vi "通知路由使用时间结束.vi"(7 "ACOM":string="A%d:COM%d", 11 "RF_Now":T1) -> ()   [LabVIEW 2011]
uses:
  Global/SeverGlobal.vi
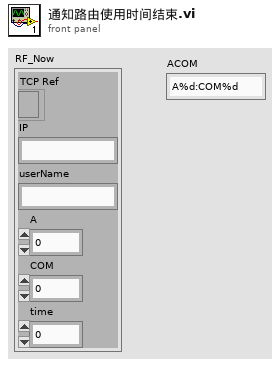
[diagram p1: front panel]
types:
  T1 = cluster{"TCP Ref":refnum<k5>, "IP":string, "userName":string, "A":u16, "COM":u16, "time":u32}
  T2 = cluster{"TCP Ref":refnum<k5>, "Broadcast":refnum<k5>, "IP":string, "port":u16, "userName":string, "passWord":string, "authority":string}[]
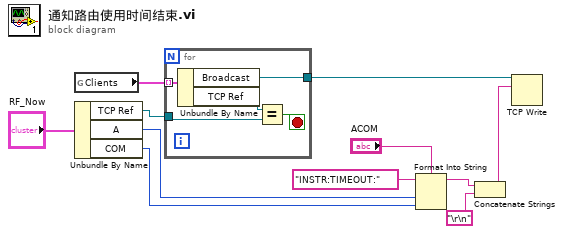
[diagram p0: block diagram]
diagram:
  n1 = global read "SeverGlobal.vi" "Clients"() -> (w9:T2)
  n2 = Unbundle By Name("RF_Now") -> ("TCP Ref"=w10:refnum<k5>, "A"=w2:u16, "COM"=w1:u16)
  n3 = for {
    tunnel: w9 -> [w16] mode=indexing
    tunnel: w10 -> [w14]
    tunnel: [w12] -> w11
    stop <- w13 stop-if-true
    n4 = Unbundle By Name(w16) -> ("Broadcast"=w12:refnum<k5>, "TCP Ref"=w15:refnum<k5>)
    n5 = Equal?(x=w15, y=w14) -> (x = y?=w13:bool)
  }
  n6 = Format Into String(format string="ACOM", initial string="INSTR:TIMEOUT:" ("data in"), w2, w1) -> (resulting string=w5:string)  [unwired: 1 in, 1 out]
  n7 = Concatenate Strings(w5, "\r\n") -> (w3:string)
  n8 = TCP Write(connection ID=w11, data in=w3) -> ()  [unwired: 2 in, 3 out]
